vi "DAQmx - Get Accele Task Infor-某型振动实验台测试系统.vi"(8 "error in (no error)":errorcluster, 11 "Accele":T1[](array[typedef])) -> (0 "error out":errorcluster, 3 "PXI-4498 Task":T1[](array[typedef]))   [LabVIEW 2011]
doc: "索引出所选振动通道信息"
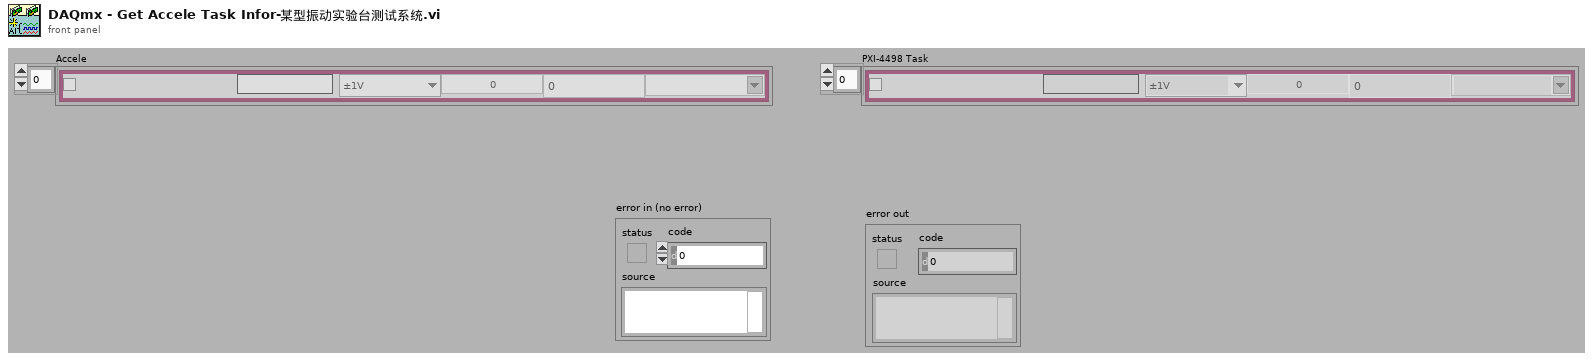
[diagram p1: front panel]
types:
  T1 = typedef "Acceleration Channel Config_Ctrls-某型振动实验台测试系统.ctl" = cluster{"Enable":bool, "Name":string, "range":enum16{"±1V", "±5V"}, "SensValue":dbl, "PhysicalName":string, "off":dbl, "Sensunits":string}
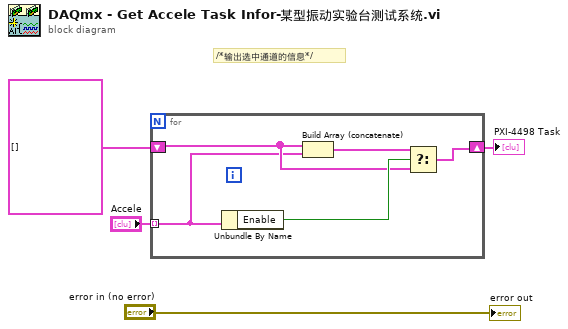
[diagram p0: block diagram]
diagram:
  # "/*输出选中通道的信息*/"
  n1 = for {
    shift-right: [w7] -> w3
    shift-left: T1[] [] -> [w6]
    tunnel: "Accele" -> [w5] mode=indexing
    n2 = Unbundle By Name(w5) -> ("Enable"=w8:bool)
    n3 = Build Array (concatenate)(w6, w5) -> (w9:T1[])
    n4 = Select(t=w9, s=w8, f=w6) -> (s? t:f=w7:T1[])
  }
  "PXI-4498 Task" <- w3
  "error out" <- "error in (no error)"
